vi "Homework_3.vi"() -> ()   [LabVIEW 2011]
uses:
  <vilib>/imath/engines/lvmath/Plug In/_Char/NIMS_CH_character datatype.ctl
  <vilib>/imath/engines/lvmath2/RunTimeEngine/NodeEndStatement/NIMS_NodeEndStatement_Output.vi
  <instcachedir>/0/NIMS_NodeEndStatement_Output_53EC0D466D134D7ABD903AC30B43404B.lvgen/NIMS_NodeEndStatement_Output_53EC0D466D134D7ABD903AC30B43404B_001.vi
  <vilib>/imath/engines/lvmath2/RunTimeEngine/ErrorHandling/NIMS_Finalize Error.vi
  <vilib>/imath/engines/lvmath2/RunTimeEngine/Managers/WorkSpace/UID Generator.vi
  <vilib>/imath/engines/lvmath2/RunTimeEngine/Managers/SymbolTable/Clear UID.vi
  <vilib>/imath/engines/lvmath2/RunTimeEngine/BuiltInFunctions/figure/NIMS_figure(I32).vi
  <vilib>/imathl/engines/lvmath/Functions/Error Handling/Create Error.vi
  <vilib>/imath/engines/lvmath2/RunTimeEngine/BuiltInFunctions/hold/NIMS_hold(Enums).vi
  <vilib>/imath/engines/lvmath2/RunTimeEngine/BuiltInFunctions/plot/NIMS_plot(RM, RM, Str).vi
  <vilib>/imath/engines/lvmath/Plug In/_Char/NIMS_CH_Character RV to String.vi
  <vilib>/imath/engines/lvmath2/RunTimeEngine/BuiltInFunctions/legend/NIMS_legend(Str).vi
  <vilib>/imath/engines/lvmath2/RunTimeEngine/Managers/SymbolTable/NIMS_WorkSpace.lvlib
panel:
  out "XY Graph":cluster{dbl[], dbl[]}[](graph)
  in  "Initial Velocity(v)":dbl
  in  "Initial Position(x)":dbl
  in  "Run Time(sec)":dbl=3.0
  in  "Time Step(sec)":dbl=0.01
  in  "Natural Frequency":dbl=25.0
  in  "Damping\nCoeffiencent":dbl=0.12
  in  "Frequency":dbl=38.0
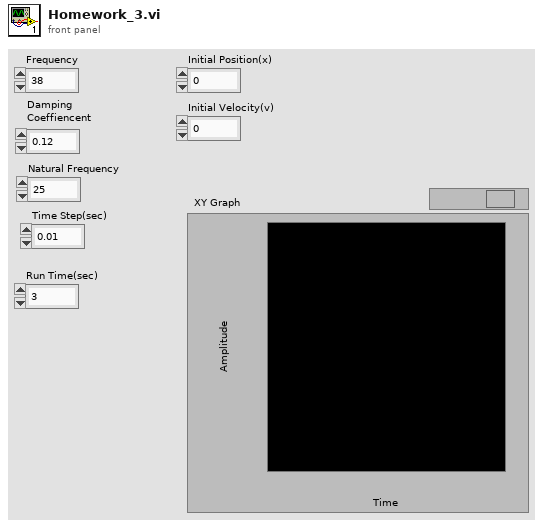
[diagram p1: front panel]
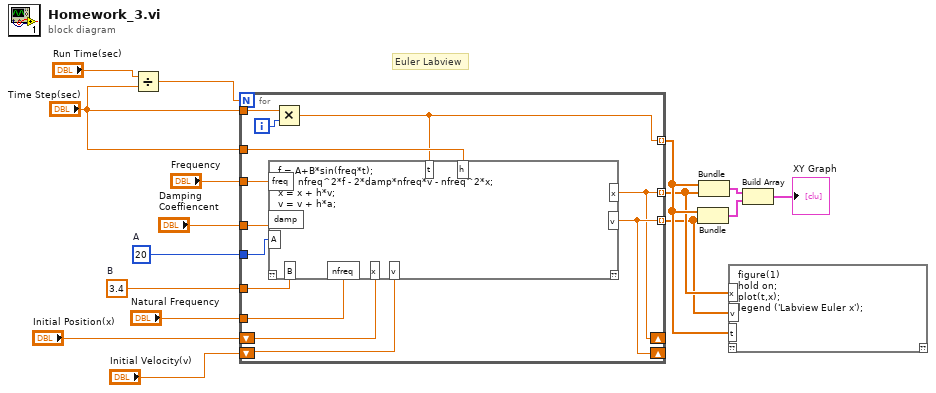
[diagram p0: block diagram]
diagram:
  w10 = 3.4  # B
  w11 = 20  # A
  # "Euler Labview"
  n1 = Divide(x="Run Time(sec)", y="Time Step(sec)") -> (x/y=w15:dbl)
  n2 = for {
    N: w15 -> [_]
    tunnel: "Frequency" -> [w29]
    tunnel: "Natural Frequency" -> [w28]
    tunnel: "Damping\nCoeffiencent" -> [w27]
    tunnel: w11 -> [w26]
    tunnel: "Time Step(sec)" -> [w25]
    tunnel: w10 -> [w24]
    tunnel: "Time Step(sec)" -> [w20]
    tunnel: [w18] -> w2 mode=indexing
    tunnel: [w19] -> w1 mode=indexing
    shift-right: [w18] -> _
    shift-left: "Initial Position(x)" -> [w22]
    shift-right: [w19] -> _
    shift-left: "Initial Velocity(v)" -> [w23]
    tunnel: [w17] -> w3 mode=indexing
    i -> [w21]
    n3 = Multiply(x=w20, y=w21) -> (x*y=w17:dbl)
    n4 = mathscript code="f = A+B*sin(freq*t);\na = nfreq^2*f - 2*damp*nfreq*v - nfreq^2*x; \nx = x + h*v;\nv = v + h*a;"("t"=w17, "h"=w25, "A"=w26, "B"=w24, "freq"=w29, "nfreq"=w28, "x"=w22, "v"=w23, "damp"=w27) -> ("x"=w18:dbl, "v"=w19:dbl)  [unwired: 1 in, 1 out]
  }
  n5 = Bundle(w3, w1) -> (w5:cluster{dbl[], dbl[]})  [unwired: 1 in]
  n6 = Bundle(w3, w2) -> (w6:cluster{dbl[], dbl[]})  [unwired: 1 in]
  n7 = mathscript code="figure(1)\nhold on;\nplot(t,x);\nlegend ('Labview Euler x');"("x"=w2, "v"=w1, "t"=w3) -> ()  [unwired: 1 in, 1 out]
  n8 = Build Array(w6, w5) -> (→"XY Graph":cluster{dbl[], dbl[]}[])
